vi "Ventile bei CG schalten.vi"   [LabVIEW 2020, in "CalGas Aufschaltung.lvlib"]
uses:
  CalGas Aufschaltung.lvlib
  FGV CalGas Aktionen.ctl
  Auswahl Aufschaltpunkt.ctl
  Auswahl Analysator.ctl
types:
  T1 = typedef "CalGas Aufschaltung.lvlib/Auswahl Analysator.ctl" = enum16{"FT-IR", "FID", "PMA", "PMA/FID/FT-IR"}
  T2 = typedef "CalGas Aufschaltung.lvlib/Auswahl Aufschaltpunkt.ctl" = enum16{"über Filterblock", "Analysator direkt", "über PNS"}
  T3 = typedef "CalGas Aufschaltung.lvlib/FGV CalGas Aktionen.ctl" = enum16{"lesen", "Def.CalGas", "Aufschaltung CalGas", "laden", "speichern", "KAL extrahieren"}
  T4 = typedef "CalGas Aufschaltung.lvlib/Aufschaltung CalGas.ctl" = cluster{"Kalibriergas":T5, "Aufschaltpunkt":T2, "Analysator":T1}
  T5 = typedef "Auswahlfeld.ctl" = u16
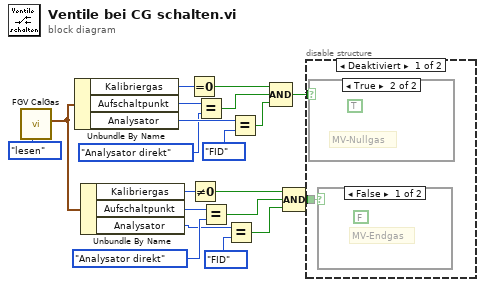
[diagram p0: block diagram]
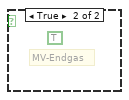
[diagram p2: hidden frame]
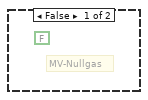
[diagram p3: hidden frame]
diagram:
  n1 = call "FGV CalGas.vi"("Aktionen"=FGV_CalGas_Aktionen."lesen") -> ("Aufschaltung CalGas"=w18:T4)  [unwired: 7 in, 3 out]
  n2 = Unbundle By Name(w18) -> ("Kalibriergas"=w6:T5, "Aufschaltpunkt"=w2:T2, "Analysator"=w4:T1)
  n3 = Unbundle By Name(w18) -> ("Kalibriergas"=w19:T5, "Aufschaltpunkt"=w17:T2, "Analysator"=w15:T1)
  n4 = Equal To 0?(x=w6) -> (x = 0?=w7:bool)
  n5 = Not Equal To 0?(x=w19) -> (x != 0?=w20:bool)
  n6 = Equal?(x=w2, y=Auswahl_Aufschaltpunkt."Analysator direkt") -> (x = y?=w8:bool)
  n7 = Equal?(x=w17, y=Auswahl_Aufschaltpunkt."Analysator direkt") -> (x = y?=w13:bool)
  n8 = Equal?(x=w15, y=Auswahl_Analysator."FID") -> (x = y?=w12:bool)
  n9 = Equal?(x=w4, y=Auswahl_Analysator."FID") -> (x = y?=w9:bool)
  n10 = Compound Arithmetic op=AND(w7, w8, w9) -> (w10:bool)
  n11 = Compound Arithmetic op=AND(w20, w13, w12) -> (w11:bool)
  n12 = disable-structure shown="Deaktiviert" {
    disable-tunnel: w11 -> [w22 _]
    disable-tunnel: w10 -> [w21 _]
    frame Disabled {
      n13 = case shown="True" w21 {
        frame False {
          (unwired) FALSE ("Zustand")
          # "MV-Nullgas"
        }
        frame True {
          (unwired) TRUE ("Zustand")
          # "MV-Nullgas"
        }
      }
      n14 = case shown="False" w22 {
        frame False {
          (unwired) FALSE ("Zustand")
          # "MV-Endgas"
        }
        frame True {
          (unwired) TRUE ("Zustand")
          # "MV-Endgas"
        }
      }
    }
    frame Enabled {
    }
  }
